vi "AI eredmények.vi"(8 "error in (no error)":errorcluster, 10 "data":dbl[][](array[numeric]), 11 "Message Queues":T1) -> (0 "error out":errorcluster)   [LabVIEW 2014]
uses:
  support/Message Queue/All Message Queues.ctl
  support/Message Queue/Message Cluster.ctl
  Analog Input Cluster.ctl
  Analog Result Cluster.ctl
  support/Message Queue/Lossy Enqueue Message (Single).vi
  support/Message Queue/Message Queue.lvlib
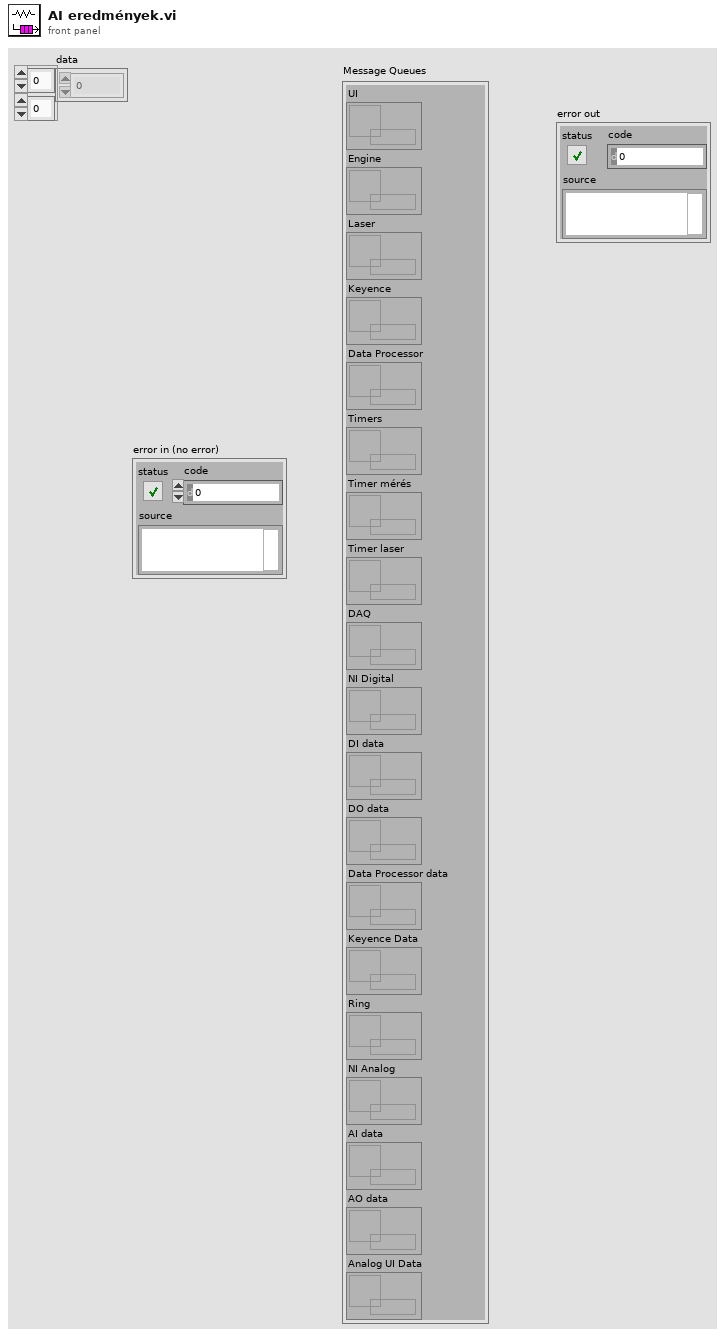
[diagram p1: front panel]
types:
  T1 = typedef "Message Queue.lvlib/All Message Queues.ctl" = cluster{"UI":refnum<queue>, "Engine":refnum<queue>, "Laser":refnum<queue>, "Keyence":refnum<queue>, "Data Processor":refnum<queue>, "Timers":refnum<queue>, "Timer mérés":refnum<queue>, "Timer laser":refnum<queue>, "DAQ":refnum<queue>, "NI Digital":refnum<queue>, "DI data":refnum<queue>, "DO data":refnum<queue>, "Data Processor data":refnum<queue>, "Keyence Data":refnum<queue>, "Ring":refnum<queue>, "NI Analog":refnum<queue>, "AI data":refnum<queue>, "AO data":refnum<queue>, "Analog UI Data":refnum<queue>}
  T2 = typedef "Analog Input Cluster.ctl" = cluster{"NI-6221":cluster{"Sensor":dbl, "Uref":dbl, "Temperature":dbl, "Uisol":dbl, "NTC":dbl, "U48":dbl, "U15":dbl}, "Analog Result":T3, "AI engedélyezés":bool, "dU":dbl[]}
  T3 = typedef "Analog Result Cluster.ctl" = cluster{"Szenzor ellenállás":dbl, "NTC ellenállás":dbl, "Szigetelési ellenállás":dbl, "Hõmérséklet":dbl, "48V":dbl, "15V":dbl, "Elvárt NTC ellenállás":dbl, "Számolt NTC hõmérséklet":dbl}
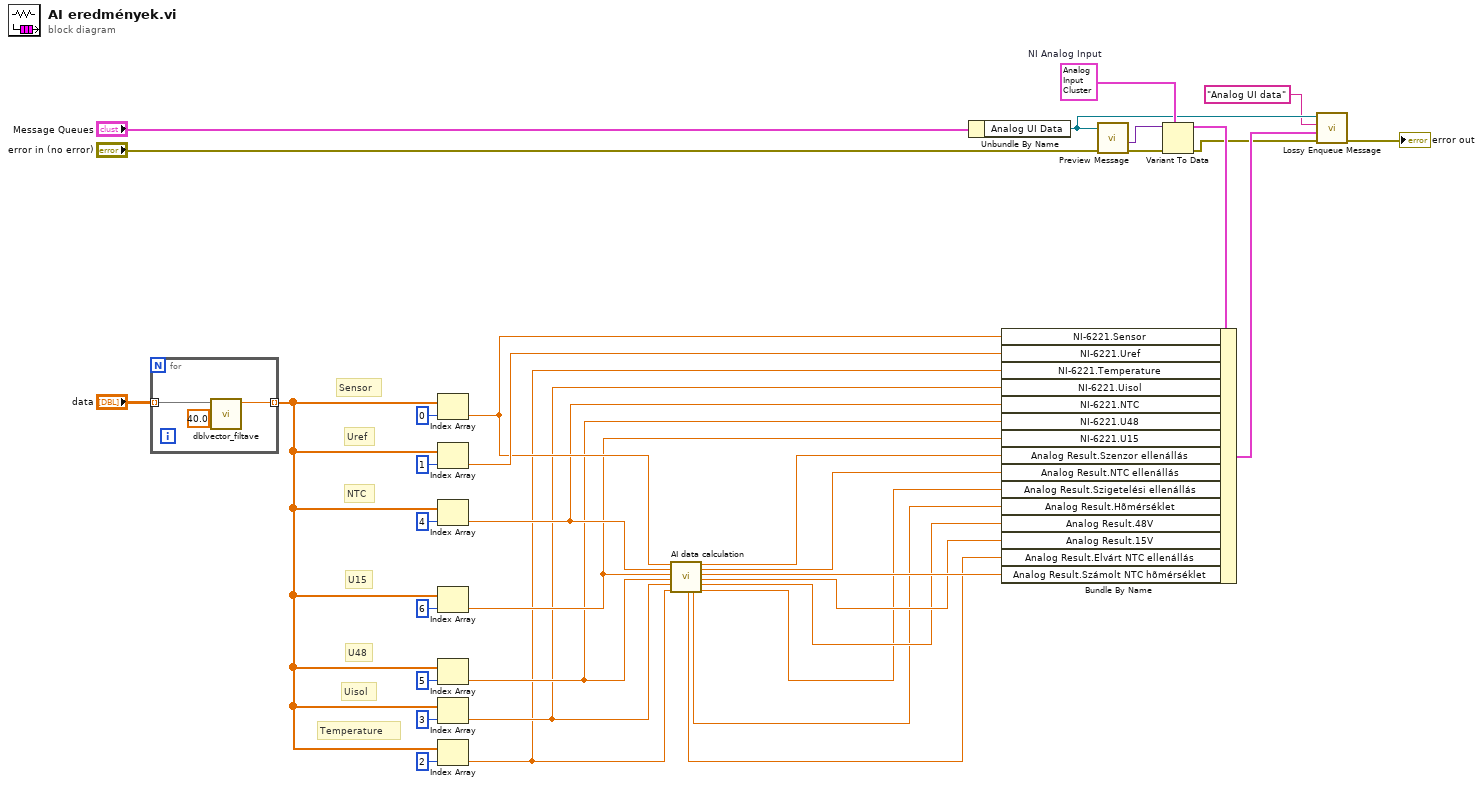
[diagram p0: block diagram]
diagram:
  w33 = T2 {"NI-6221"={"Sensor"=0.0, "Uref"=0.0, "Temperature"=0.0, "Uisol"=0.0, "NTC"=0.0, "U48"=0.0, "U15"=0.0}, "Analog Result"={"Szenzor ellenállás"=0.0, "NTC ellenállás"=0.0, "Szigetelési ellenállás"=0.0, "Hõmérséklet"=0.0, "48V"=0.0, "15V"=0.0, "Elvárt NTC ellenállás"=0.0, "Számolt NTC hõmérséklet"=0.0}, "AI engedélyezés"=FALSE, "dU"=[]}  # NI Analog Input
  # "Temperature"
  # "Uisol"
  # "U48"
  # "U15"
  # "NTC"
  # "Uref"
  # "Sensor"
  n1 = for {
    tunnel: "data" -> [w37] mode=indexing
    tunnel: [w36] -> w16 mode=indexing
    n2 = call "dblvector_filtave.vi"("Eldobandó [%]"=40.0, "Mérési adatok"=w37) -> ("Szûrt átlag"=w36:dbl)  [unwired: 9 in]
  }
  n3 = Index Array(array=w16, index=0) -> (element=w14:dbl)
  n4 = Index Array(array=w16, index=1 ("index (row)")) -> (element=w15:dbl)
  n5 = Index Array(array=w16, index=4 ("index (row)")) -> (element=w12:dbl)
  n6 = Index Array(array=w16, index=6 ("index (row)")) -> (element=w11:dbl)
  n7 = Index Array(array=w16, index=5 ("index (row)")) -> (element=w10:dbl)
  n8 = Index Array(array=w16, index=3 ("index (row)")) -> (element=w9:dbl)
  n9 = Index Array(array=w16, index=2 ("index (row)")) -> (element=w8:dbl)
  n10 = call "AI data calculation.vi"("Sensor raw"=w14, "NTC raw"=w12, "U15 raw"=w11, "U48 raw"=w10, "Isol raw"=w9, "Temp raw"=w8) -> ("NTC ellenállás elvárt"=w1:dbl, "Hõmérséklet"=w2:dbl, "Sensor ellenállás"=w13:dbl, "NTC ellenállás"=w7:dbl, "NTC Hõmérséklet számolt"=w6:dbl, "15V"=w5:dbl, "48V"=w4:dbl, "Szigetelési ellenállás"=w3:dbl)  [unwired: 6 in]
  n11 = Unbundle By Name("Message Queues") -> ("Analog UI Data"=w21:refnum<queue>)
  n12 = call "Preview Message.vi"("error in (no error)"="error in (no error)", "Message Queue"=w21) -> ("error out"=w34:errorcluster, "Message Data"=w35:variant)  [unwired: 5 in, 3 out]
  n13 = Variant To Data(error in=w34, type=w33, Variant=w35) -> (data=w31:T2, error out=w20:errorcluster)
  n14 = Bundle By Name(cluster=w31, "NI-6221.Sensor"=w14, "NI-6221.Uref"=w15, "NI-6221.Temperature"=w8, "NI-6221.Uisol"=w9, "NI-6221.NTC"=w12, "NI-6221.U48"=w10, "NI-6221.U15"=w11, "Analog Result.Szenzor ellenállás"=w13, "Analog Result.NTC ellenállás"=w7, "Analog Result.Szigetelési ellenállás"=w3, "Analog Result.Hõmérséklet"=w2, "Analog Result.48V"=w4, "Analog Result.15V"=w5, "Analog Result.Elvárt NTC ellenállás"=w1, "Analog Result.Számolt NTC hõmérséklet"=w6) -> (w22:T2)
  n15 = call-poly "Lossy Enqueue Message.vi"("error in (no error)"=w20, "Message Data"=w22, "Message"="Analog UI data", "Message Queue"=w21) -> ("error out"=→"error out":errorcluster)  [unwired: 6 in, 1 out]
